vi "Array to String.vi"(7 "Strings? (F)":bool, 11 "JSON Strings":string[](array[string])) -> (3 "JSON Array String":string)   [LabVIEW 2018, in "JSON.lvlib"]
uses:
  JSON.lvlib
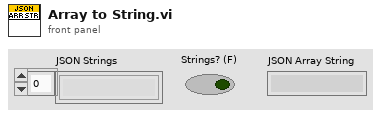
[diagram p1: front panel]
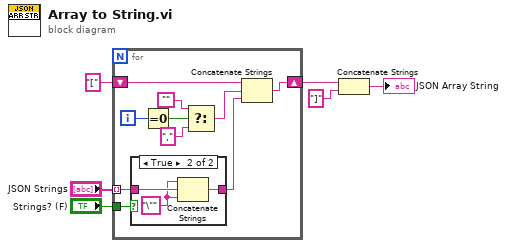
[diagram p0: block diagram]
diagram:
  n1 = for {
    shift-right: [w10] -> w5
    shift-left: "[" -> [w12]
    tunnel: "JSON Strings" -> [w8] mode=indexing
    tunnel: "Strings? (F)" -> [w9]
    i -> [w16]
    n2 = case shown="True" w9 {
      tunnel: w8 -> [w17 w20]
      tunnel: [w17 w18] -> w7
      frame False {
      }
      frame True {
        w19 = "\"" ("string")
        n3 = Concatenate Strings(w19, w20, w19) -> (w18:string)
      }
    }
    n4 = Equal To 0?(x=w16) -> (x = 0?=w15:bool)
    n5 = Select(t="", s=w15, f=",") -> (s? t:f=w11:string)
    n6 = Concatenate Strings(w12, w11, w7) -> (w10:string)
  }
  n7 = Concatenate Strings(w5, "]" ("string")) -> (→"JSON Array String":string)
